vi "RealtimeData.vi"(1 "新增数据":dbl[](array[numeric]), 2 "action":enum16{"initialize", "append", "get"}(ring), 5 "曲线名":string[](array[string]), 7 "曲线标尺":i32[](array[numeric]), 9 "开始时间":timestamp, 11 "时间间隔":dbl, 12 "新增备注":string) -> (3 "数据":dbl[][](array[numeric]), 6 "曲线名":string[](array[string]), 8 "曲线标尺":i32[](array[numeric]), 10 "开始时间":timestamp, 14 "备注":string[](array[string]), 15 "时间间隔":dbl)   [LabVIEW 2020]
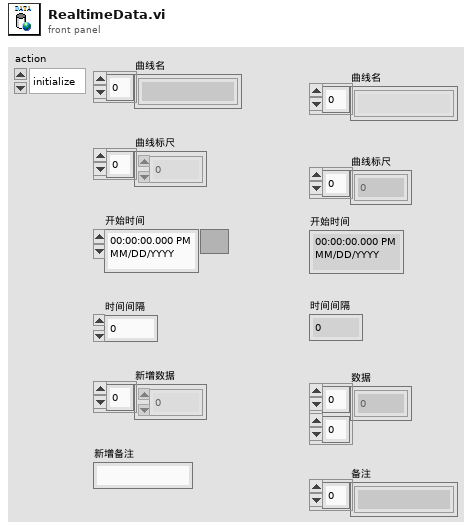
[diagram p1: front panel]
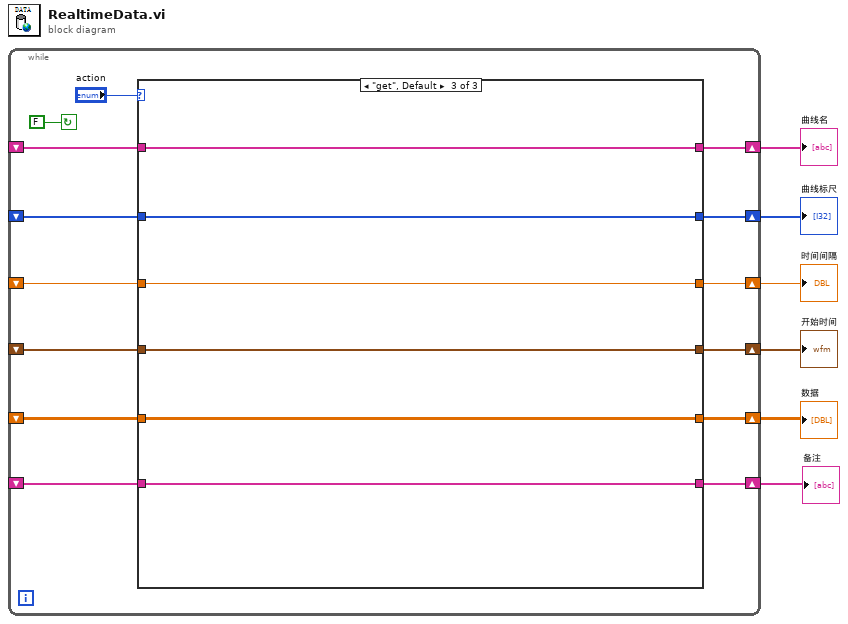
[diagram p0: block diagram]
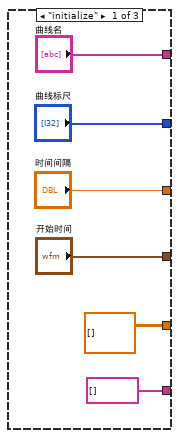
[diagram p2: hidden frame]
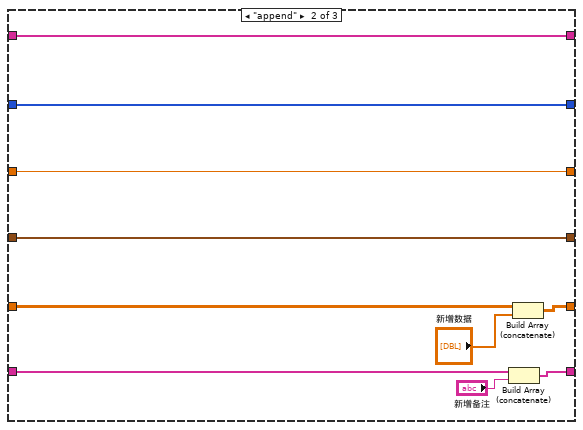
[diagram p3: hidden frame]
diagram:
  n1 = while {
    shift-right: [w18] -> w6
    shift-left: _ -> [w14]
    shift-right: [w17] -> w5
    shift-left: _ -> [w13]
    shift-right: [w16] -> w4
    shift-left: _ -> [w12]
    shift-right: [w15] -> w3
    shift-left: _ -> [w11]
    shift-right: [w10] -> w2
    shift-left: _ -> [w8]
    shift-right: [w9] -> w1
    shift-left: _ -> [w7]
    stop <- FALSE continue-if-true
    n2 = case shown="\"get\", Default" "action" {
      tunnel: ["曲线名" w36 w42] -> w18
      tunnel: ["曲线标尺" w35 w41] -> w17
      tunnel: ["时间间隔" w34 w40] -> w16
      tunnel: ["开始时间" w33 w39] -> w15
      tunnel: w14 -> [_ w36 w42]
      tunnel: w13 -> [_ w35 w41]
      tunnel: w12 -> [_ w34 w40]
      tunnel: w11 -> [_ w33 w39]
      tunnel: [dbl[][] [] ("数据") w32 w38] -> w10
      tunnel: [string[] [] ("备注") w29 w37] -> w9
      tunnel: w8 -> [_ w31 w38]
      tunnel: w7 -> [_ w28 w37]
      frame "initialize" {
      }
      frame "append" {
        n3 = Build Array (concatenate)(w28, "新增备注") -> (w29:string[])
        n4 = Build Array (concatenate)(w31, "新增数据") -> (w32:dbl[][])
      }
      frame "get", Default {
      }
    }
  }
  "曲线标尺" <- w5
  "时间间隔" <- w4
  "曲线名" <- w6
  "开始时间" <- w3
  "数据" <- w2
  "备注" <- w1
